vi "USB_DAQ__EEPROM_Test_Single_Byte_Read_24C32.vi"() -> ()   [LabVIEW 2022 SP3]
panel:
  in  "Page.Address.0":u8 format="%02x"
  out "Page.ACK.0":bool
  out "Addr.ACK.2":bool
  out "Data.Byte.Read":u8 format="%02x"
  out "RunTime.ms":u32
  in  "Page.Address.1":u8 format="%02x"
  out "Page.ACK.1":bool
  out "Addr.ACK.1":bool
  in  "24C32.Address":u8=87 format="%02x"
  in  "Read":bool
  # "EEPROM 24C32 READ"
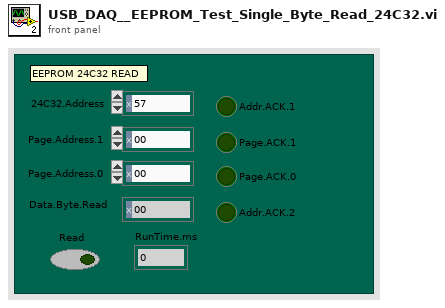
[diagram p1: front panel]
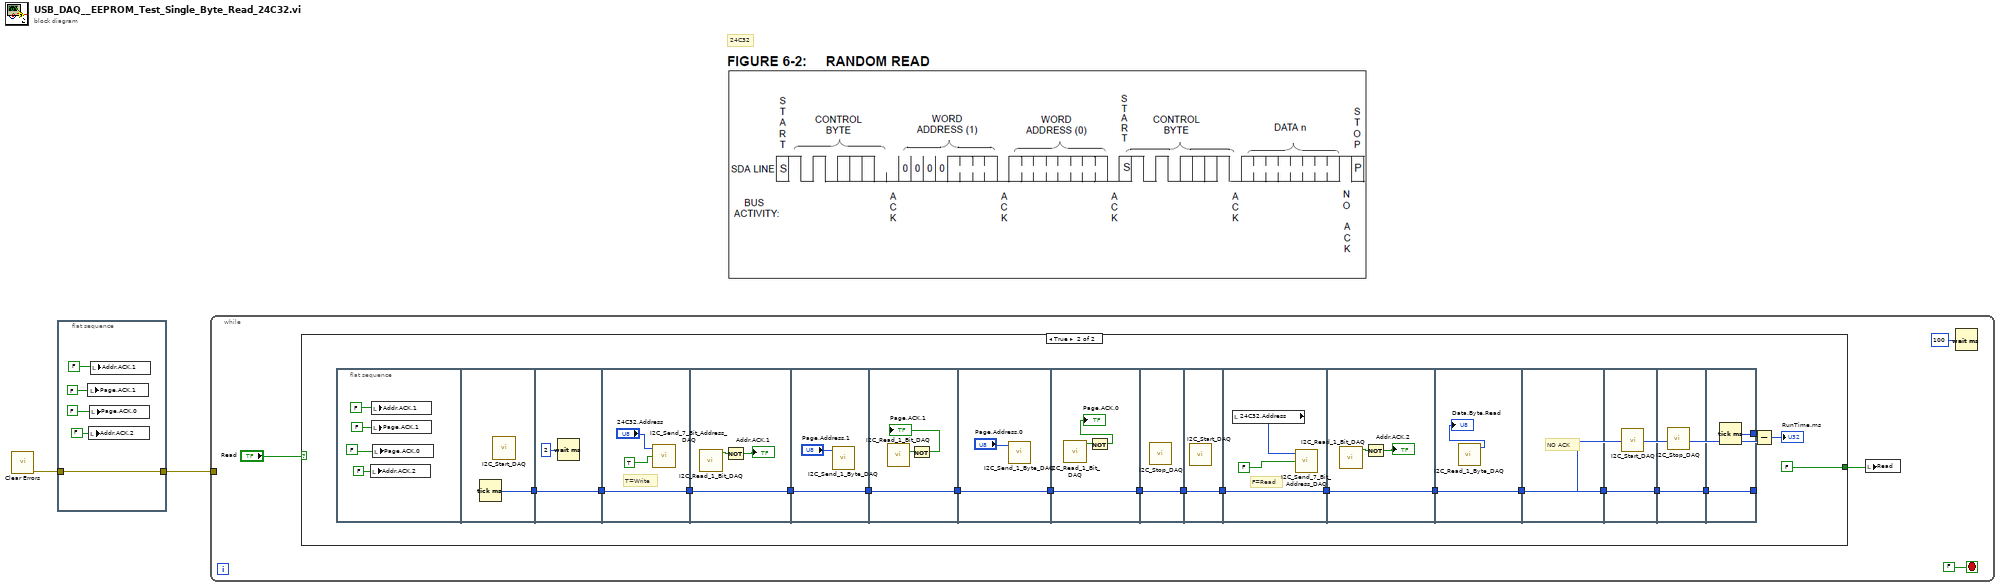
[diagram p0: block diagram]
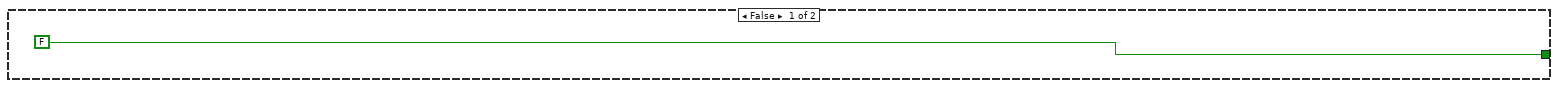
[diagram p2: hidden frame]
diagram:
  # "24C32"
  n1 = call <vilib>:"Clear Errors.vi"() -> ("error out"=w1:errorcluster)  [unwired: 6 in, 1 out]
  n2 = flat-sequence {
    tunnel: w1 -> [w7]
    tunnel: [w7] -> w2
    frame #0 {
      n3 = local write "Page.ACK.1"(FALSE ("TX.ACK")) -> ()
      n4 = local write "Addr.ACK.2"(FALSE ("Addr.ACK.2")) -> ()
      n5 = local write "Page.ACK.0"(FALSE ("Page.ACK.0")) -> ()
      n6 = local write "Addr.ACK.1"(FALSE ("ACK_OK")) -> ()
    }
  }
  n7 = while {
    tunnel: w2 -> [_]
    stop <- FALSE stop-if-true
    n8 = case shown="True" "Read" {
      tunnel: [FALSE ("Test") FALSE ("Test")] -> w8
      frame False {
      }
      frame True {
        n9 = flat-sequence {
          tunnel: [w37] -> w23
          tunnel: [w38] -> w24
          tunnel: w23 -> [w38]
          tunnel: [w40] -> w25
          tunnel: w24 -> [w40]
          tunnel: [w43] -> w26
          tunnel: w25 -> [w43]
          tunnel: [w46] -> w27
          tunnel: w26 -> [w46]
          tunnel: [w48] -> w15
          tunnel: w27 -> [w48]
          tunnel: w15 -> [w52]
          tunnel: [w52] -> w14
          tunnel: w14 -> [w55]
          tunnel: [w55] -> w13
          tunnel: w13 -> [w56]
          tunnel: [w56] -> w17
          tunnel: w17 -> [w57]
          tunnel: [w57] -> w16
          tunnel: w16 -> [w60]
          tunnel: [w60] -> w19
          tunnel: w19 -> [w63]
          tunnel: [w63] -> w18
          tunnel: [w65] -> w28
          tunnel: w18 -> [w65]
          tunnel: [w66] -> w29
          tunnel: w28 -> [w66]
          tunnel: [w67] -> w30
          tunnel: w29 -> [w67]
          tunnel: [w68] -> w31
          tunnel: w30 -> [w68]
          tunnel: w31 -> [w69]
          tunnel: [w70] -> w21
          tunnel: [w69] -> w20
          frame #0 {
            n10 = local write "Addr.ACK.2"(FALSE ("Addr.ACK.2")) -> ()
            n11 = local write "Addr.ACK.1"(FALSE ("ACK_OK")) -> ()
            n12 = local write "Page.ACK.1"(FALSE ("TX.ACK")) -> ()
            n13 = local write "Page.ACK.0"(FALSE ("Page.ACK.0")) -> ()
          }
          frame #1 {
            n14 = Tick Count (ms)() -> (millisecond timer value=w37:u32)
            n15 = call "I2C_Start_DAQ.vi"() -> ()  [unwired: 6 in]
          }
          frame #2 {
            n16 = Wait (ms)(milliseconds to wait=u32 2) -> ()  [unwired: 1 out]
          }
          frame #3 {
            # "T=Write"
            n17 = call "I2C_Send_7_Bit_Address_DAQ.vi"("Write or Read?"=TRUE, "Receiver_7_Bit_Address"="24C32.Address") -> ()  [unwired: 1 in]
          }
          frame #4 {
            n18 = call "I2C_Read_1_Bit_DAQ.vi"() -> ("RX_Bit_Out"=w45:bool)  [unwired: 2 in]
            n19 = Not(x=w45) -> (.not. x?=→"Addr.ACK.1":bool)
          }
          frame #5 {
            n20 = call "I2C_Send_1_Byte_DAQ.vi"("Byte_To_Send"="Page.Address.1") -> ()  [unwired: 2 in]
          }
          frame #6 {
            n21 = call "I2C_Read_1_Bit_DAQ.vi"() -> ("RX_Bit_Out"=w50:bool)  [unwired: 2 in]
            n22 = Not(x=w50) -> (.not. x?=→"Page.ACK.1":bool)
          }
          frame #7 {
            n23 = call "I2C_Send_1_Byte_DAQ.vi"("Byte_To_Send"="Page.Address.0") -> ()  [unwired: 2 in]
          }
          frame #8 {
            n24 = call "I2C_Read_1_Bit_DAQ.vi"() -> ("RX_Bit_Out"=w54:bool)  [unwired: 2 in]
            n25 = Not(x=w54) -> (.not. x?=→"Page.ACK.0":bool)
          }
          frame #9 {
            n26 = call "I2C_Stop_DAQ.vi"() -> ()  [unwired: 6 in]
          }
          frame #10 {
            n27 = call "I2C_Start_DAQ.vi"() -> ()  [unwired: 6 in]
          }
          frame #11 {
            # "F=Read"
            n28 = local read "24C32.Address"() -> (w58:u8)
            n29 = call "I2C_Send_7_Bit_Address_DAQ.vi"("Write or Read?"=FALSE, "Receiver_7_Bit_Address"=w58) -> ()  [unwired: 1 in]
          }
          frame #12 {
            n30 = call "I2C_Read_1_Bit_DAQ.vi"() -> ("RX_Bit_Out"=w62:bool)  [unwired: 2 in]
            n31 = Not(x=w62) -> (.not. x?=→"Addr.ACK.2":bool)
          }
          frame #13 {
            n32 = call "I2C_Read_1_Byte_DAQ.vi"() -> ("Byte.Data.Read"=→"Data.Byte.Read":u8)  [unwired: 2 in]
          }
          frame #14 {
            # "NO ACK"
          }
          frame #15 {
            n33 = call "I2C_Start_DAQ.vi"() -> ()  [unwired: 6 in]
          }
          frame #16 {
            n34 = call "I2C_Stop_DAQ.vi"() -> ()  [unwired: 6 in]
          }
          frame #17 {
            n35 = Tick Count (ms)() -> (millisecond timer value=w70:u32)
          }
        }
        n36 = Subtract(x=w21, y=w20) -> (x-y=→"RunTime.ms":u32)
      }
    }
    n37 = local write "Read"(w8) -> ()
    n38 = Wait (ms)(milliseconds to wait=u32 100) -> ()  [unwired: 1 out]
  }
